vi "UDP Remote Port Test.vi"() -> ()   [LabVIEW 2014, in "ESP8266 WiFi Wrapper.lvlib"]
uses:
  <vilib>/Aledyne-TSXperts/Arduino Compatible Compiler for LabVIEW/addons/ESP8266 WiFi Wrapper/ESP8266 WiFi Wrapper.lvlib
panel:
  out "Remote Host Port":u16
  out "Error Out":errorcluster
  in  "Error In":errorcluster
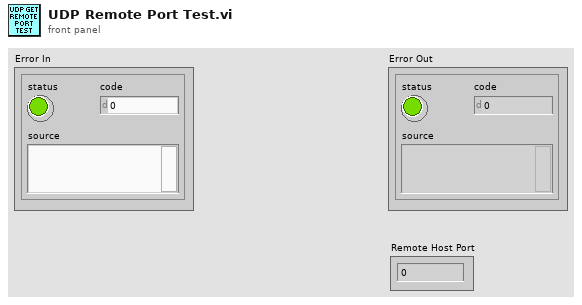
[diagram p1: front panel]
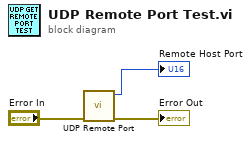
[diagram p0: block diagram]
diagram:
  n1 = call <vilib>:"UDP Remote Port.vi"("Error In"="Error In") -> ("Error Out"=→"Error Out":errorcluster, "Port of remote host"=→"Remote Host Port":u16)  [unwired: 9 in]
